vi "981 Manipulator Init.vi"(1 "error in":errorcluster) -> (0 "error out":errorcluster)   [LabVIEW 2014]
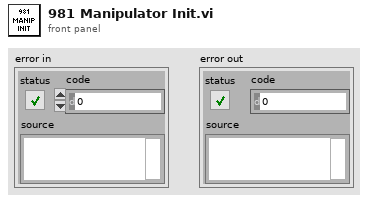
[diagram p1: front panel]
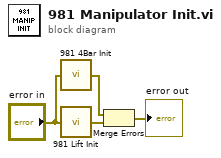
[diagram p0: block diagram]
diagram:
  n1 = call "981 4Bar Init.vi"("error in (no error)"="error in") -> ("error out"=w1:errorcluster)
  n2 = call "981 Lift Init.vi"("error in (no error)"="error in") -> ("error out"=w2:errorcluster)
  n3 = Merge Errors(w1, w2) -> (→"error out":errorcluster)
